vi "GUI_Arduino.vi"() -> ()   [LabVIEW 2013]
uses:
  <vilib>/Instr/_visa.llb/VISA Configure Serial Port (Instr).vi
panel:
  out "Arduino Data":string
  in  "Stop":bool
  out "Error":errorcluster
  in  "Angle":string
  in  "Mode":bool
  in  "Baud Rate":u32=9600
  in  "Port":refnum<visa-resource-name>
  # "Arduino Interface"
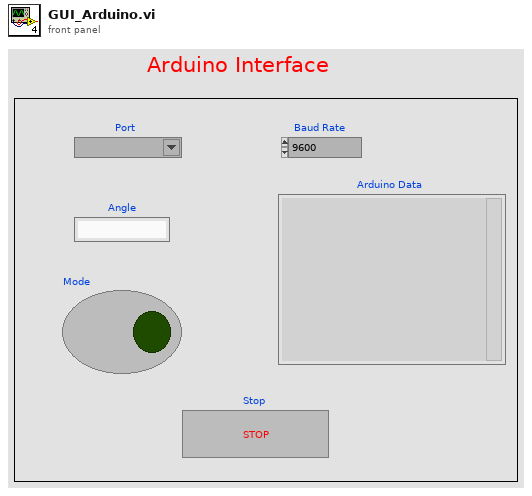
[diagram p1: front panel]
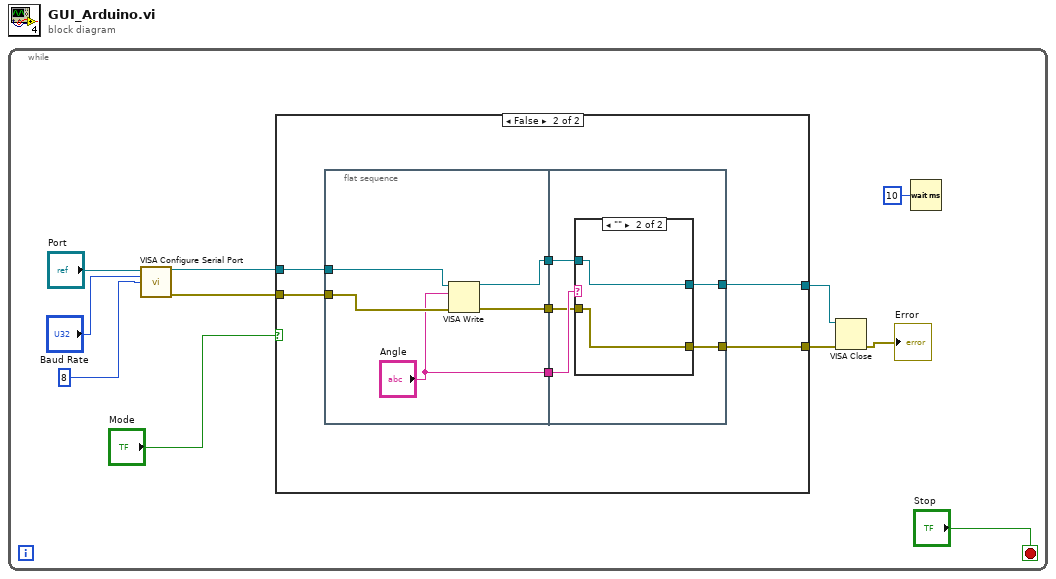
[diagram p0: block diagram]
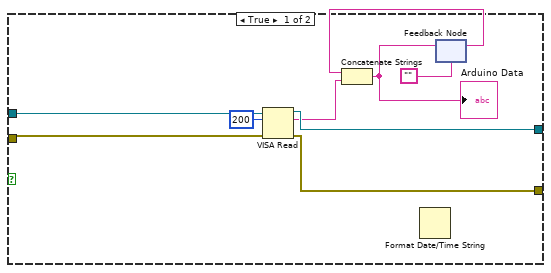
[diagram p2: hidden frame]
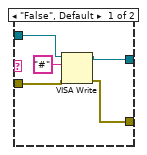
[diagram p3: hidden frame]
diagram:
  n1 = while {
    stop <- "Stop" stop-if-true
    n2 = call-poly "VISA Configure Serial Port"("VISA resource name"="Port", "baud rate (9600)"="Baud Rate", "data bits (8)"=u16 8) -> ("VISA resource name out"=w1:refnum<visa-resource-name>, "error out"=w2:errorcluster)  [unwired: 11 in]
    n3 = case shown="False" "Mode" {
      tunnel: w1 -> [w18 w27]
      tunnel: [w19 w21] -> w10
      tunnel: [w20 w22] -> w11
      tunnel: w2 -> [w17 w26]
      frame True {
        n4 = VISA Read(VISA resource name=w18, byte count=u32 200, error in (no error)=w17) -> (VISA resource name out=w20:refnum<visa-resource-name>, read buffer=w15:string, error out=w19:errorcluster)  [unwired: 1 out]
        n5 = Format Date/Time String() -> ()  [unwired: 3 in, 1 out]
        n6 = feedback #1("") -> (w14:string)
        n7 = Concatenate Strings(w14, w15) -> (w13:string)
        "Arduino Data" <- w13
        n8 = feedback-in #1(w13) -> ()
      }
      frame False {
        n9 = flat-sequence {
          tunnel: w27 -> [w32]
          tunnel: w26 -> [w31]
          tunnel: ["Angle"] -> w25
          tunnel: [w29] -> w24
          tunnel: [w28] -> w23
          tunnel: w25 -> [w37]
          tunnel: w24 -> [w36]
          tunnel: w23 -> [w35]
          tunnel: [w34] -> w22
          tunnel: [w33] -> w21
          frame #0 {
            n10 = VISA Write(VISA resource name=w32, write buffer="Angle", error in (no error)=w31) -> (VISA resource name out=w29:refnum<visa-resource-name>, error out=w28:errorcluster)  [unwired: 1 out]
          }
          frame #1 {
            n11 = case shown="\"\"" w37 {
              tunnel: w36 -> [w41 w44]
              tunnel: w35 -> [w40 w43]
              tunnel: [w39 w44] -> w34
              tunnel: [w38 w43] -> w33
              frame "False", Default {
                n12 = VISA Write(VISA resource name=w41, write buffer="#", error in (no error)=w40) -> (VISA resource name out=w39:refnum<visa-resource-name>, error out=w38:errorcluster)  [unwired: 1 out]
              }
              frame "" {
              }
            }
          }
        }
      }
    }
    n13 = VISA Close(VISA resource name=w11, error in (no error)=w10) -> (error out=→"Error":errorcluster)
    n14 = Wait (ms)(milliseconds to wait=u32 10) -> ()  [unwired: 1 out]
  }
